vi "MHX Tube Wall Temperature.vi"(6 "Sec Ave Temperature (K)":dbl, 9 "Pri Ave Temperature (K)":dbl, 10 "MHX Shell h":dbl, 11 "MHX Tube h":dbl) -> (3 "MHX Tube Wall Temperature (K)":dbl)   [LabVIEW 2019]
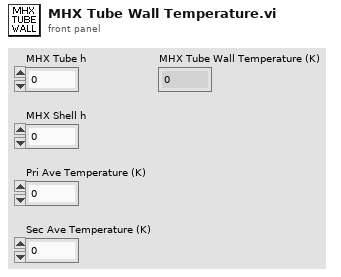
[diagram p1: front panel]
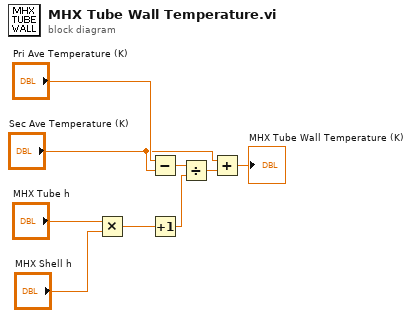
[diagram p0: block diagram]
diagram:
  n1 = Multiply(x="MHX Tube h", y="MHX Shell h") -> (x*y=w7:dbl)
  n2 = Subtract(x="Pri Ave Temperature (K)", y="Sec Ave Temperature (K)") -> (x-y=w3:dbl)
  n3 = Increment(x=w7) -> (x+1=w6:dbl)
  n4 = Divide(x=w3, y=w6) -> (x/y=w2:dbl)
  n5 = Add(x="Sec Ave Temperature (K)", y=w2) -> (x+y=→"MHX Tube Wall Temperature (K)":dbl)
